vi "Read THD.vi"(8 "error in (no error)":errorcluster, 11 "Universal Power Meter in":refnum<class "Universal Power Meter.lvclass">) -> (0 "error out":errorcluster, 2 "THD?":bool, 3 "Universal Power Meter out":refnum<class "Universal Power Meter.lvclass">)   [LabVIEW 2013, in "Universal Power Meter.lvlib" / "Universal Power Meter.lvclass"]
uses:
  Universal Power Meter.lvclass
  Universal Power Meter.lvclass/Universal Power Meter.ctl
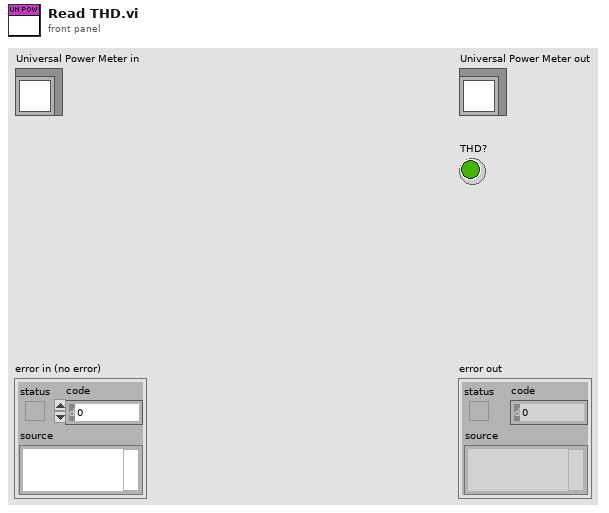
[diagram p1: front panel]
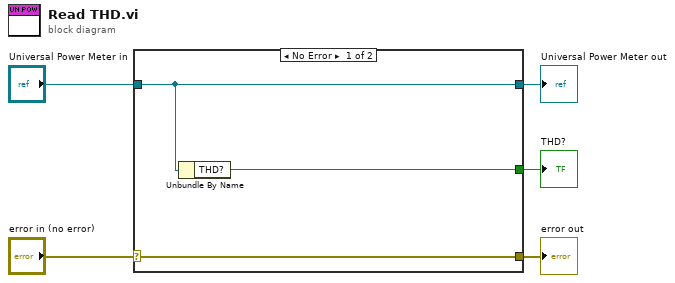
[diagram p0: block diagram]
diagram:
  n1 = case shown="No Error" "error in (no error)" {
    selector: "error in (no error)" -> [w8 w9]
    tunnel: [w8 w9] -> w4
    tunnel: [w7 w10] -> w2
    tunnel: "Universal Power Meter in" -> [w7 w10]
    tunnel: [w6 _] -> w1
    frame No Error {
      n2 = Unbundle By Name(w7) -> ("THD?"=w6:bool)
    }
    frame Error {
    }
  }
  "error out" <- w4
  "Universal Power Meter out" <- w2
  "THD?" <- w1
